vi "Compile Communication Config.vi"(8 "error in (no error)":errorcluster, 11 "Device Ref in":T1 format="%.0x") -> (0 "error out":errorcluster, 2 "Communication Configuration":T2, 3 "Device Ref out":T1 format="%.0x")   [LabVIEW 2017, in "Routing and Faulting System Explorer.lvlib"]
uses:
  Routing and Faulting System Explorer.lvlib
  Shared/Communication Configuration.ctl
  <vilib>/NI Veristand/Custom Device API/Custom Device Item Ref.ctl
  Shared/Routing and Faulting Shared.lvlib
  <vilib>/NI VeriStand/Custom Device API/Custom Device API.lvlib
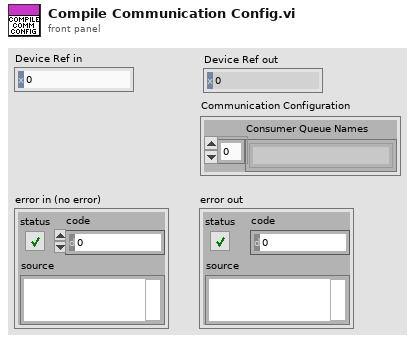
[diagram p1: front panel]
types:
  T1 = typedef "Custom Device API.lvlib/Custom Device Item Ref.ctl" = u64
  T2 = typedef "Routing and Faulting Shared.lvlib/Communication Configuration.ctl" = cluster{"Consumer Queue Names":string[]}
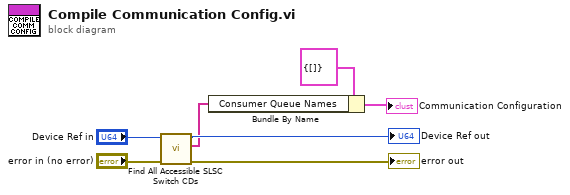
[diagram p0: block diagram]
diagram:
  n1 = call "Find All Accessible SLSC Switch CDs.vi"("error in (no error)"="error in (no error)", "Custom device ref in"="Device Ref in") -> ("error out"=→"error out":errorcluster, "SLSC Switch CD Paths"=w2:string[], "Custom device ref out"=→"Device Ref out":T1)  [unwired: 7 in]
  n2 = Bundle By Name(cluster=T2 {"Consumer Queue Names"=[]} ("Communication Configuration 2"), "Consumer Queue Names"=w2) -> (→"Communication Configuration":T2)
